vi "Read Processing.vi"(8 "error in (no error)":errorcluster, 11 "CV-Main in":refnum<class "CV-Main.lvclass">) -> (0 "error out":errorcluster, 2 "Processing":refnum<notifier>, 3 "CV-Main out":refnum<class "CV-Main.lvclass">)   [LabVIEW 2013, in "CameraVision.lvlib" / "CV-Main.lvclass"]
uses:
  CV-Main.lvclass
  CV-Main.lvclass/CV-Main.ctl
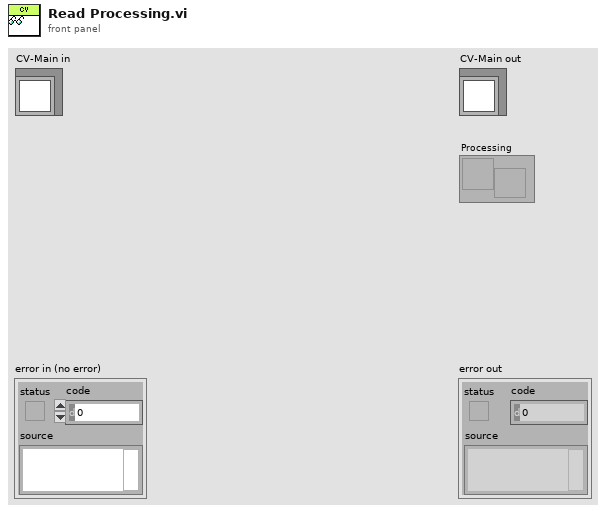
[diagram p1: front panel]
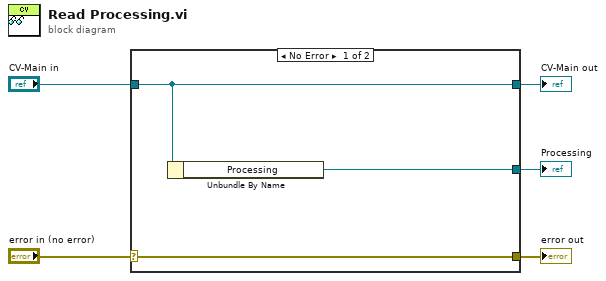
[diagram p0: block diagram]
diagram:
  n1 = case shown="No Error" "error in (no error)" {
    selector: "error in (no error)" -> [w8 w9]
    tunnel: [w8 w9] -> w4
    tunnel: [w7 w10] -> w2
    tunnel: "CV-Main in" -> [w7 w10]
    tunnel: [w6 _] -> w1
    frame No Error {
      n2 = Unbundle By Name(w7) -> ("Processing"=w6:refnum<notifier>)
    }
    frame Error {
    }
  }
  "error out" <- w4
  "CV-Main out" <- w2
  "Processing" <- w1
